vi "Remove Queue.vi"(9 "Queue":refnum<queue>, 11 "Channel Data In":T1) -> (3 "Channel Data":T1)   [LabVIEW 2022 SP3, in "Flex.lvlib"]
uses:
  Flex.lvlib
  Channel Data.ctl
  Element Info.ctl
  Element.ctl
  Event Data.ctl
  Queue Data.ctl
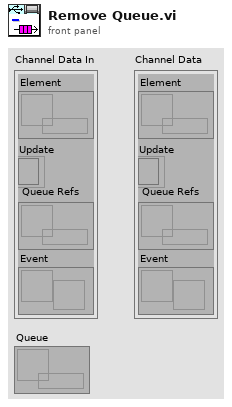
[diagram p1: front panel]
types:
  T1 = typedef "Flex.lvlib/Channel Data.ctl" = cluster{"Element":refnum<data-value>, "Update":refnum<k4>, "Queue Refs":refnum<data-value>, "Event":refnum<user-event>}
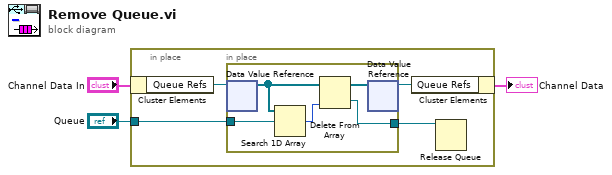
[diagram p0: block diagram]
diagram:
  n1 = in-place {
    in-place-border: "Queue" -> [w5]
    n2 = in-place-cluster #1("Channel Data In") -> ("Queue Refs"=w7:refnum<data-value>)
    n3 = in-place {
      in-place-border: w5 -> [w12]
      in-place-border: [w8] -> w4
      n4 = in-place-dvr #2(w7) -> (w11:refnum<queue>[])  [unwired: 1 out]
      n5 = Search 1D Array(1D array=w11, element=w12) -> (index of element=w10:i32)  [unwired: 1 in]
      n6 = Delete From Array(array=w11, index=w10) -> (deleted portion=w8:refnum<queue>, array with subset deleted=w9:refnum<queue>[])  [unwired: 1 in]
      n7 = in-place-dvr #2(w9) -> (w6:refnum<data-value>)  [unwired: 1 out]
    }
    n8 = in-place-cluster #1("Queue Refs"=w6) -> (→"Channel Data":T1)
    n9 = Release Queue(queue=w4) -> ()  [unwired: 2 in, 3 out]
  }
